vi "FPGA.vi"() -> ()   [LabVIEW 2016]
uses:
  <vilib>/EmbeddedDisplay/Hitachi HD44780/Common/Control/8bit connection map.ctl
  <vilib>/EmbeddedDisplay/Hitachi HD44780/Common/HD44780 Common.lvlib
  <vilib>/EmbeddedDisplay/Hitachi HD44780/FPGA/HD44780 FPGA.lvlib
  <vilib>/EmbeddedDisplay/Hitachi HD44780/FPGA/Internal/LCD Command.vi
  <vilib>/EmbeddedDisplay/Hitachi HD44780/Common/Control/lcd command cluster.ctl
  <vilib>/eio/EIONode/EIONode.xnode
  <vilib>/rvi/eio/common/nirviEmuTemplateMethod_errors.vi
  <vilib>/Platform/TimedLoop/XDataNode/wakeup.ctl
  <vilib>/Platform/TimedLoop/XDataNode/XDNodeRunTimeDep.lvlib
  <vilib>/Platform/TimedLoop/XDataNode/nitl_modes.ctl
  <vilib>/Platform/TimedLoop/XDataNode/timing_clust.ctl
  <vilib>/Platform/TimedLoop/XDataNode/XDataNode.xnode
  <vilib>/EmbeddedDisplay/Hitachi HD44780/FPGA/Public/Command Handler (8 Bits).vi
panel:
  out "Position":i16
  in  "Reset":bool
  out "E-Stop":bool
  in  "PWM":bool
  in  "LCD Command":T1={"device index (-1)"=-1, "operation (0)"=0}
  # "Encoder Loop"
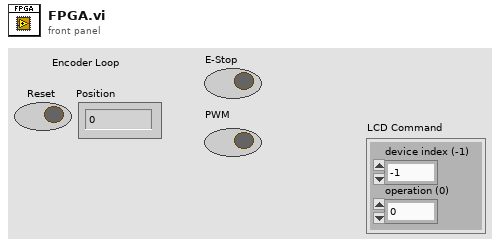
[diagram p1: front panel]
types:
  T1 = typedef "HD44780 Common.lvlib/lcd command cluster.ctl" = cluster{"device index (-1)":i8, "operation (0)":u32}
  T2 = typedef "XDNodeRunTimeDep.lvlib/timing_clust.ctl" = cluster{"Expected End [f-1]":u64, "Actual End [f-1]":u64, "Finished Late? [f-1]":bool, "Expected End [i-1]":u64, "Actual End [i-1]":u64, "Finished Late? [i-1]":bool, "Expected Start [i]":u64, "Actual Start [i]":u64, "Expected Start [f]":u64, "Actual Start [f]":u64, "Source Name":string, "Structure Name":string, "Period":i64, "Deadline":i64, "Offset":i64, "Start":i64, "Priority":i32, "Timeout":i32, "Mode":T3, "Wakeup Reason":T4, "Error":errorcluster, "Source Type":string, "Secondary Source Type":string, "Global End Time":u64, "Global Start Time":u64, "Frame Duration":u64, "Iteration Duration":u64, "Assigned CPU":i32, "I/O Scan Engine Mode":u32}
  T3 = typedef "XDNodeRunTimeDep.lvlib/nitl_modes.ctl" = enum32{"No Change", "Process missed periods, maintain original phase", "Discard missed periods, maintain original phase", "Process missed periods, ignore original phase", "Discard missed periods, ignore original phase"}
  T4 = typedef "XDNodeRunTimeDep.lvlib/wakeup.ctl" = enum32{"Normal", "Aborted", "Asynchronous wakeup", "Timing source error", "Timed loop error", "Timeout"}
  T5 = typedef "HD44780 Common.lvlib/8bit connection map.ctl" = cluster{"RS":refnum<k21>, "R/W":refnum<k21>, "E1":refnum<k21>, "E2":refnum<k21>, "DB0":refnum<k21>, "DB1":refnum<k21>, "DB2":refnum<k21>, "DB3":refnum<k21>, "DB4":refnum<k21>, "DB5":refnum<k21>, "DB6":refnum<k21>, "DB7":refnum<k21>}
  T6 = cluster{"device index (-1)":i8, "operation (0)":u32}
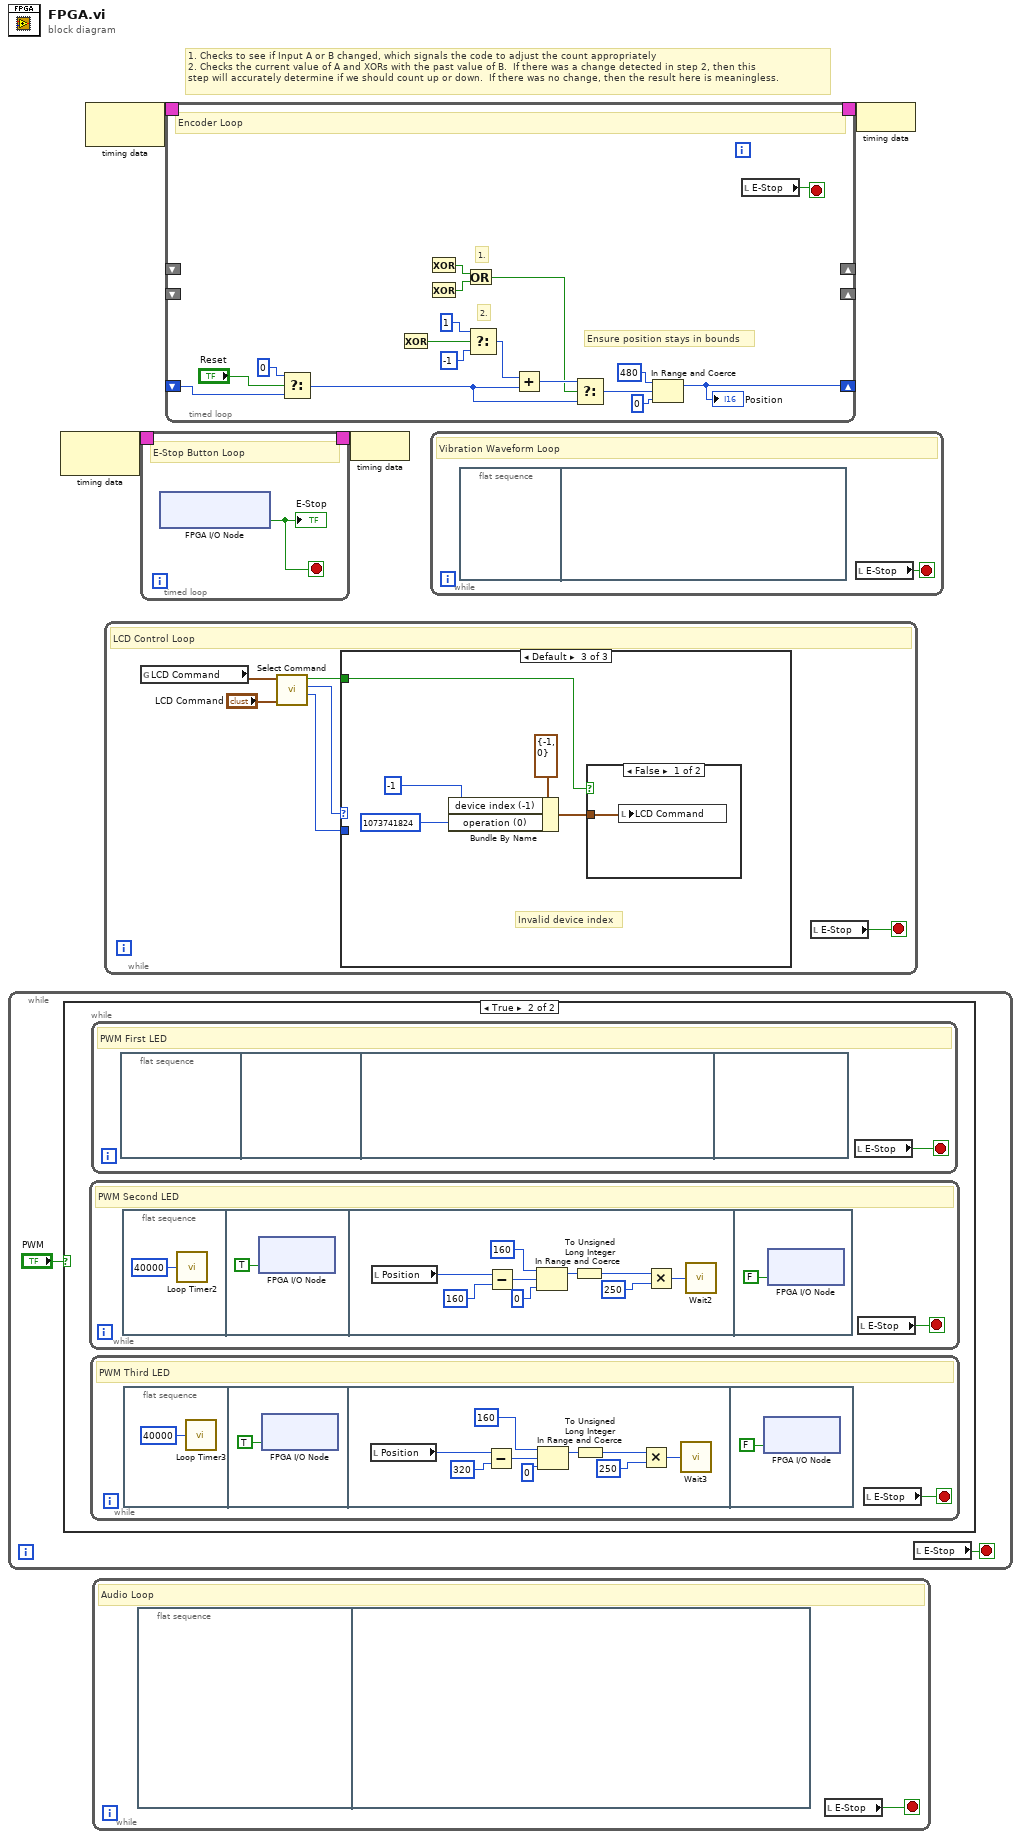
[diagram p0: block diagram]
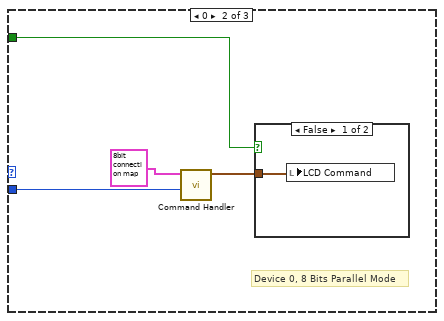
[diagram p3: hidden frame]
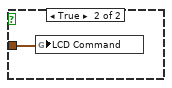
[diagram p4: hidden frame]
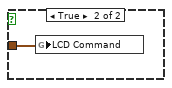
[diagram p5: hidden frame]
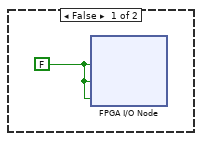
[diagram p6: hidden frame]
diagram:
  # "1. Checks to see if Input A or B changed, which signals the code to adjust the count appropriately\n2. Checks the current value of A and XORs with the past value of B.  If there was a change detected in step 2, then this \nstep will accurately determine if we should count up or down.  If there was no change, then the result here is meaningless."
  n1 = while {
    stop <- w5 stop-if-true
    n2 = case shown="True" "PWM" {
      frame False {
        w7 = FALSE ("DIO4")
        n3 = xnode "FPGA I/O Node"("LED1"=w7, "LED2"=w7, "LED3"=w7) -> ()  [unwired: 3 in, 3 out]
      }
      frame True {
        n4 = while {
          stop <- w21 stop-if-true
          # "PWM Second LED"
          n5 = flat-sequence {
            frame #0 {
              n6 = call "Loop Timer2"("Count(Ticks)"=u32 40000) -> ()  [unwired: 1 out]
            }
            frame #1 {
              n7 = xnode "FPGA I/O Node"("LED2"=TRUE ("DIO5")) -> ()  [unwired: 1 in, 1 out]
            }
            frame #2 {
              n8 = local read "Position"() -> (w24:i16)
              n9 = Subtract(x=w24, y=i16 160) -> (x-y=w28:i16)
              n10 = In Range and Coerce(upper limit=i16 160, x=w28, lower limit=i16 0) -> (coerced(x)=w26:i16)  [unwired: 1 out]
              n11 = To Unsigned Long Integer(number=w26) -> (unsigned 32bit integer=w25:u32)
              n12 = Multiply(x=w25, y=u32 250) -> (x*y=w29:u32)
              n13 = call "Wait2"("Count(Ticks)"=w29) -> ()  [unwired: 1 out]
            }
            frame #3 {
              n14 = xnode "FPGA I/O Node"("LED2"=FALSE ("DIO5")) -> ()  [unwired: 1 in, 1 out]
            }
          }
          n15 = local read "E-Stop"() -> (w21:bool)
        }
        n16 = while {
          stop <- w8 stop-if-true
          # "PWM Third LED"
          n17 = flat-sequence {
            frame #0 {
              n18 = call "Loop Timer3"("Count(Ticks)"=u32 40000) -> ()  [unwired: 1 out]
            }
            frame #1 {
              n19 = xnode "FPGA I/O Node"("LED3"=TRUE ("DIO5")) -> ()  [unwired: 1 in, 1 out]
            }
            frame #2 {
              n20 = local read "Position"() -> (w11:i16)
              n21 = Subtract(x=w11, y=i16 320) -> (x-y=w14:i16)
              n22 = In Range and Coerce(upper limit=i16 160, x=w14, lower limit=i16 0) -> (coerced(x)=w13:i16)  [unwired: 1 out]
              n23 = To Unsigned Long Integer(number=w13) -> (unsigned 32bit integer=w12:u32)
              n24 = Multiply(x=w12, y=u32 250) -> (x*y=w16:u32)
              n25 = call "Wait3"("Count(Ticks)"=w16) -> ()  [unwired: 1 out]
            }
            frame #3 {
              n26 = xnode "FPGA I/O Node"("LED3"=FALSE ("DIO5")) -> ()  [unwired: 1 in, 1 out]
            }
          }
          n27 = local read "E-Stop"() -> (w8:bool)
        }
        n28 = while {
          stop <- w34 stop-if-true
          # "PWM First LED"
          n29 = flat-sequence {
            frame #0 {
            }
            frame #1 {
            }
            frame #2 {
            }
            frame #3 {
            }
          }
          n30 = local read "E-Stop"() -> (w34:bool)
        }
      }
    }
    n31 = local read "E-Stop"() -> (w5:bool)
  }
  n32 = node-c288() -> (w4:T2)  [unwired: 1 in]
  n33 = node-c288() -> (w2:T2)  [unwired: 1 in]
  n34 = while {
    stop <- w35 stop-if-true
    # "Audio Loop"
    n35 = flat-sequence {
      frame #0 {
      }
      frame #1 {
      }
    }
    n36 = local read "E-Stop"() -> (w35:bool)
  }
  n37 = while {
    stop <- w36 stop-if-true
    # "LCD Control Loop"
    n38 = global read "LCD Command.vi" "LCD Command"() -> (w37:T6)
    n39 = call <vilib>:"Select Command.vi"("Host LCD Command"="LCD Command", "FPGA LCD Command"=w37) -> ("operation"=w39:u32, "device index"=w40:i8, "FPGA? True : False"=w38:bool)  [unwired: 7 in]
    n40 = case shown="Default" w40 {
      tunnel: w39 -> [_ w45 _]
      tunnel: w38 -> [_ w44 w52]
      frame -1 {
        # "IDLE State"
      }
      frame 0 {
        # "Device 0, 8 Bits Parallel Mode"
        n41 = call-poly <vilib>:"Command Handler.vi"("operation"=w45, "device connection map in"=T5 {"RS"="DIO19", "R/W"="DIO18", "E1"="DIO17", "E2"="DIO17", "DB0"="DIO20", "DB1"="DIO21", "DB2"="DIO22", "DB3"="DIO23", "DB4"="DIO24", "DB5"="DIO25", "DB6"="DIO26", "DB7"="DIO27"}) -> ("result"=w43:T6)  [unwired: 9 in]
        n42 = case shown="False" w44 {
          tunnel: w43 -> [w46 w47]
          frame False {
            n43 = local write "LCD Command"(w46) -> ()
          }
          frame True {
            n44 = global write "LCD Command.vi" "LCD Command"(w47) -> ()
          }
        }
      }
      frame Default {
        # "Invalid device index"
        n45 = Bundle By Name(cluster=T1 {"device index (-1)"=-1, "operation (0)"=0} ("LCD Command"), "device index (-1)"=i8 -1 ("LCD_device index (-1)"), "operation (0)"=u32 1073741824 ("LCD_operation (0)")) -> (w48:T1)
        n46 = case shown="False" w52 {
          tunnel: w48 -> [w53 w54]
          frame False {
            n47 = local write "LCD Command"(w53) -> ()
          }
          frame True {
            n48 = global write "LCD Command.vi" "LCD Command"(w54) -> ()
          }
        }
      }
    }
    n49 = local read "E-Stop"() -> (w36:bool)
  }
  n50 = timed-loop {
    timing: w4 -> [_]
    timing-out: [_] -> w3
    stop <- w55 stop-if-true
    # "E-Stop Button Loop"
    n51 = xnode "FPGA I/O Node"() -> ("Right Button"=w55:bool)  [unwired: 1 in, 1 out]
    "E-Stop" <- w55
  }
  n52 = timed-loop {
    shift-left: _ -> [_]
    shift-right: _ -> [_]
    shift-left: _ -> [w71]
    shift-right: [w62] -> _
    shift-left: _ -> [_]
    shift-right: _ -> [_]
    timing: w2 -> [_]
    timing-out: [_] -> w1
    stop <- w58 stop-if-true
    # "2."
    # "1."
    # "Ensure position stays in bounds"
    # "Encoder Loop"
    n53 = Select(t=i16 0, s="Reset", f=w71) -> (s? t:f=w72:i16)
    n54 = Exclusive Or() -> (0:w64:bool)  [unwired: 1 in, 1 out]
    n55 = Exclusive Or() -> (0:w66:bool)  [unwired: 2 in]
    n56 = Exclusive Or() -> (0:w67:bool)  [unwired: 1 in, 1 out]
    n57 = Or(x=w66, y=w67) -> (x .or. y?=w65:bool)
    n58 = Select(t=i16 1, s=w64, f=i16 -1) -> (s? t:f=w70:i16)
    n59 = Add(x=w70, y=w72) -> (x+y=w74:i16)
    n60 = Select(t=w74, s=w65, f=w72) -> (s? t:f=w63:i16)
    n61 = In Range and Coerce(upper limit=i16 480, x=w63, lower limit=i16 0) -> (coerced(x)=w62:i16)  [unwired: 1 out]
    "Position" <- w62
    n62 = local read "E-Stop"() -> (w58:bool)
  }
  n63 = node-c288(w3) -> ()
  n64 = while {
    stop <- w77 stop-if-true
    # "Vibration Waveform Loop"
    n65 = flat-sequence {
      frame #0 {
      }
      frame #1 {
      }
    }
    n66 = local read "E-Stop"() -> (w77:bool)
  }
  n67 = node-c288(w1) -> ()
